vi "Launch VILab.vi"   [LabVIEW 2018]
uses:
  VILab.vi
  VILab.lvlib
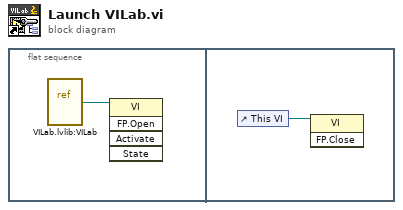
[diagram p0: block diagram]
diagram:
  n1 = flat-sequence {
    frame #0 {
      n2 = vi-ref "VILab.lvlib:VILab.vi"() -> (w1:refnum<vi>)
      n3 = invoke class="VI" method="FP.Open"(reference=w1) -> ()  [unwired: 4 in, 5 out]
    }
    frame #1 {
      n4 = control-ref of="This VI"() -> (w2:refnum<vi>)
      n5 = invoke class="VI" method="FP.Close"(reference=w2) -> ()  [unwired: 2 in, 3 out]
    }
  }
